vi "10 - Who am I.vi"() -> ()   [LabVIEW 2020]
uses:
  client/client.lvlib
panel:
  out "Display Name":string
  out "User Email":string
  out "Org RID":string
  out "User RID":string
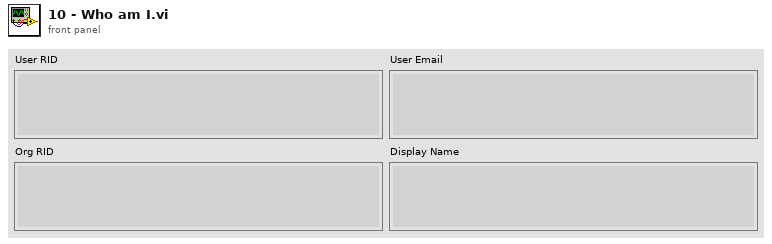
[diagram p1: front panel]
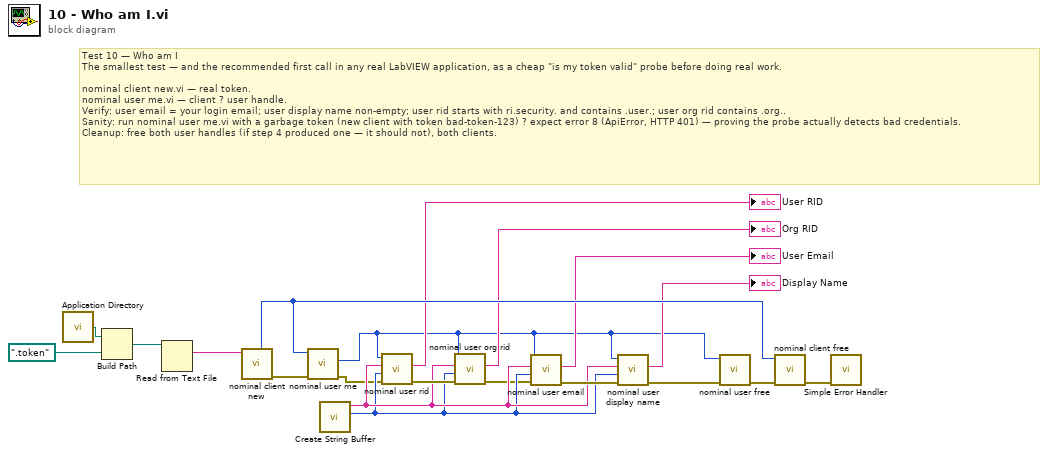
[diagram p0: block diagram]
diagram:
  # "Test 10 — Who am I\nThe smallest test — and the recommended first call in any real LabVIEW application, as a cheap \"is my token valid\" probe before doing real work.\n\nnominal client new.vi — real token.\nnominal user me.vi — client ? user handle.\nVerify: user email = your login email; user display name non-empty; user rid starts with ri.security. and contains .user.; user org rid contains .org..\nSanity: run nominal user me.vi with a garbage token (new client with token bad-token-123) ? expect error 8 (ApiError, HTTP 401) — proving the probe actually detects bad credentials.\nCleanup: free both user handles (if step 4 produced one — it should not), both clients."
  n1 = call <vilib>:"Application Directory.vi"() -> ("Application Directory"=w20:path)
  n2 = Build Path(base path=w20, name or relative path=path ".token") -> (appended path=w18:path)
  n3 = Read from Text File(file (use dialog)=w18) -> (text=w1:string)  [unwired: 3 in, 3 out]
  n4 = call "nominal client new.vi"("token"=w1) -> ("error out"=w8:errorcluster, "out_client out"=w9:i32)  [unwired: 8 in, 1 out]
  n5 = call "nominal user me.vi"("error in (no error)"=w8, "client"=w9) -> ("error out"=w11:errorcluster, "out_user out"=w2:i32)  [unwired: 7 in, 1 out]
  n6 = call "Create String Buffer.vi"() -> ("dub Buffer Size"=w13:i32, "String Buffer"=w14:string)  [unwired: 9 in, 1 out]
  n7 = call "nominal user rid.vi"("error in (no error)"=w11, "cap"=w13, "buf"=w14, "user"=w2) -> ("error out"=w16:errorcluster, "buf out"=→"User RID":string)  [unwired: 4 in, 2 out]
  n8 = call "nominal user org rid.vi"("error in (no error)"=w16, "cap"=w13, "buf"=w14, "user"=w2) -> ("error out"=w12:errorcluster, "buf out"=→"Org RID":string)  [unwired: 4 in, 2 out]
  n9 = call "nominal user email.vi"("error in (no error)"=w12, "cap"=w13, "buf"=w14, "user"=w2) -> ("error out"=w15:errorcluster, "buf out"=→"User Email":string)  [unwired: 4 in, 2 out]
  n10 = call "nominal user display name.vi"("error in (no error)"=w15, "cap"=w13, "buf"=w14, "user"=w2) -> ("error out"=w10:errorcluster, "buf out"=→"Display Name":string)  [unwired: 4 in, 2 out]
  n11 = call "nominal user free.vi"("error in (no error)"=w10, "user"=w2) -> ("error out"=w7:errorcluster)  [unwired: 8 in, 1 out]
  n12 = call "nominal client free.vi"("error in (no error)"=w7, "client"=w9) -> ("error out"=w17:errorcluster)  [unwired: 8 in, 1 out]
  n13 = call <vilib>:"Simple Error Handler.vi"("error in (no error)"=w17) -> ()  [unwired: 4 in, 5 out]
